vi "addTests.vi"(8 "error in (no error)":errorcluster, 10 "tests":refnum<class>[](array[class]), 11 "TestSuite in":refnum<class "TestSuite.lvclass">) -> (0 "error out":errorcluster, 3 "TestSuite out":refnum<class "TestSuite.lvclass">)   [LabVIEW 2013, in "TestSuite.lvclass"]
doc: "Adds 'tests' to testSuite. 'tests' can be testCase or testSuite objects (can be mixed)."
uses:
  TestSuite.lvclass
panel:
  # "JKI VI Tester for LabVIEW\nhttp://jkisoft.com/vi-tester/\nCopyright (C) 2007-2009, JKI <info@jkisoft.com>\nALL RIGHTS RESERVED"
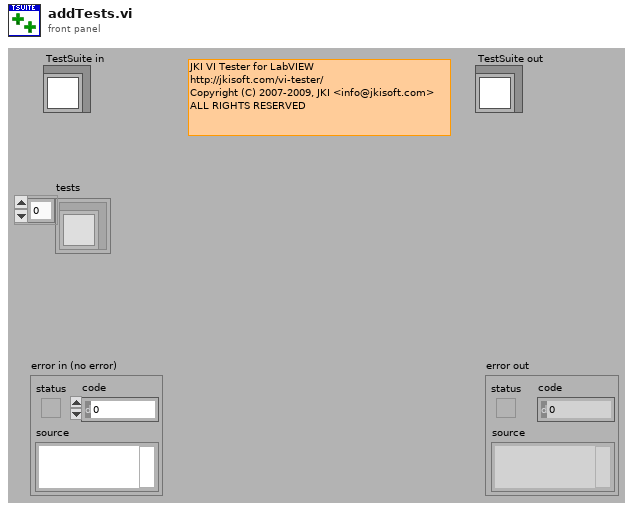
[diagram p1: front panel]
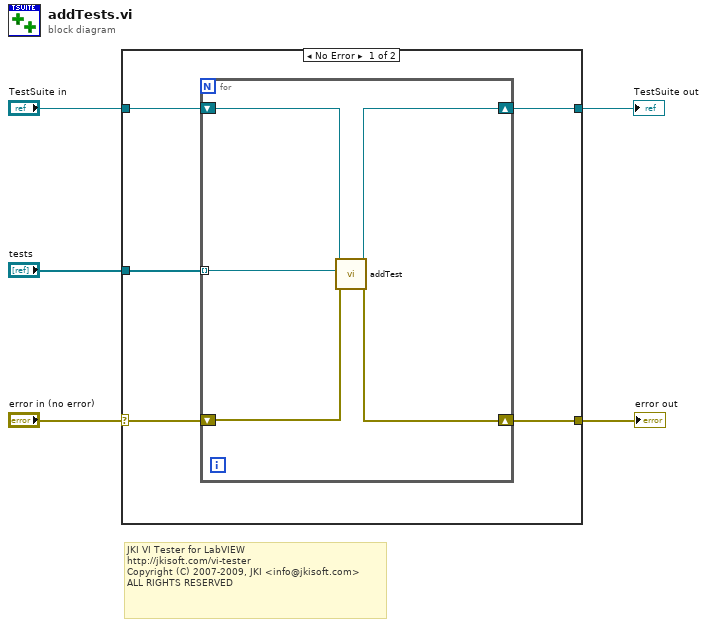
[diagram p0: block diagram]
diagram:
  # "JKI VI Tester for LabVIEW\nhttp://jkisoft.com/vi-tester\nCopyright (C) 2007-2009, JKI <info@jkisoft.com>\nALL RIGHTS RESERVED"
  n1 = case shown="No Error" "error in (no error)" {
    selector: "error in (no error)" -> [w10 w17]
    tunnel: [w7 w17] -> w4
    tunnel: [w8 w16] -> w2
    tunnel: "TestSuite in" -> [w9 w16]
    tunnel: "tests" -> [w6 _]
    frame No Error {
      n2 = for {
        shift-right: [w13] -> w8
        shift-left: w9 -> [w14]
        shift-right: [w12] -> w7
        shift-left: w10 -> [w15]
        tunnel: w6 -> [w11] mode=indexing
        n3 = call-dynamic "addTest.vi"("error in (no error)"=w15, "test"=w11, "TestSuite in"=w14) -> ("error out"=w12:errorcluster, "TestSuite out"=w13:refnum<class "TestSuite.lvclass">)  [unwired: 7 in]
      }
    }
    frame Error {
    }
  }
  "error out" <- w4
  "TestSuite out" <- w2
